vi "행복도.vi"(6 "밝기":dbl, 8 "진폭변화":dbl, 9 "잡음":dbl, 10 "역동성":dbl, 11 "템포":dbl) -> (3 "행복도":dbl format="%.2g")   [LabVIEW 2020]
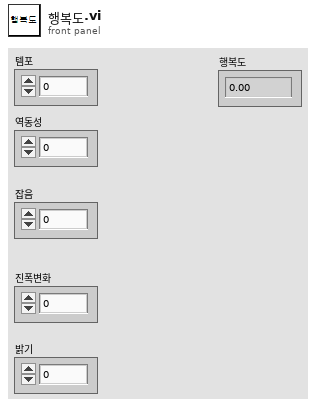
[diagram p1: front panel]
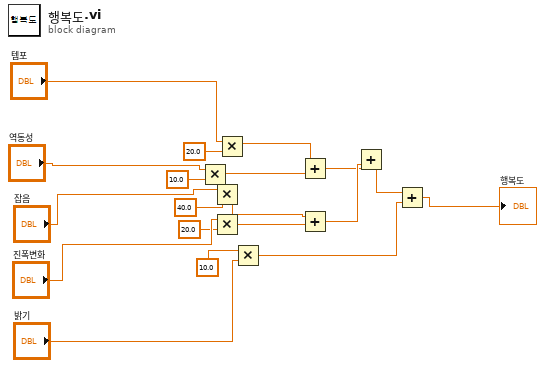
[diagram p0: block diagram]
diagram:
  n1 = Multiply(x="역동성", y=10.0) -> (x*y=w16:dbl)
  n2 = Multiply(x="잡음", y=40.0) -> (x*y=w15:dbl)
  n3 = Multiply(x="진폭변화", y=20.0) -> (x*y=w14:dbl)
  n4 = Multiply(x="템포", y=20.0) -> (x*y=w4:dbl)
  n5 = Multiply(x=10.0, y="밝기") -> (x*y=w2:dbl)
  n6 = Add(x=w4, y=w16) -> (x+y=w3:dbl)
  n7 = Add(x=w15, y=w14) -> (x+y=w13:dbl)
  n8 = Add(x=w3, y=w13) -> (x+y=w12:dbl)
  n9 = Add(x=w12, y=w2) -> (x+y=→"행복도":dbl)
